vi "Reactor.vi"() -> ()   [LabVIEW 2017]
uses:
  <vilib>/Analysis/baseanly.llb/Mean (DBL).vi
  <vilib>/Utility/file.llb/Read Delimited Spreadsheet (DBL).vi
  <vilib>/Analysis/NI_AALBase.lvlib
panel:
  in  "Flow Data?":bool=TRUE
  in  "error in (no error)":errorcluster
  in  "CTAH Set Point":sgl format="%.1f"
  in  "Mode":string(combo)
  out "Server OK":bool
  out "System Time [s]":sgl
  out "Power Output":sgl(graph)
  out "Frequency [Hz]":sgl(slide) scale=0.0..60.0
  out "Frequency [Hz]":sgl(slide) scale=0.0..60.0
  out "Frequency [Hz]":sgl(knob) scale=0.0..45.0
  out "Power [W]":sgl(slide) caption="Power Output [W]" scale=0.0..10000.0
  in  "Desired Power [W]":dbl min=0.0 max=10000.0 step=1.0 format="%.1f"
  out "WT-10":sgl format="%.1f"
  out "BT-11":sgl format="%.1f"
  out "BT-12":sgl format="%.1f"
  out "WT-13":sgl format="%.1f"
  out "CX-10":dbl format="%.1f"
  out "CX-11":dbl format="%.1f"
  out "WT-20":sgl format="%.1f"
  out "BT-21":sgl format="%.1f"
  out "WT-22":sgl format="%.1f"
  out "BT-23":sgl format="%.1f"
  out "WT-24":sgl format="%.1f"
  out "BT-25":sgl format="%.1f"
  out "WT-26":sgl format="%.1f"
  out "BT-27":sgl format="%.1f"
  out "WT-28":sgl format="%.1f"
  out "BT-29":sgl format="%.1f"
  out "BT-30":sgl format="%.1f"
  out "WT-31":sgl format="%.1f"
  out "BT-32":sgl format="%.1f"
  out "WT-33":sgl format="%.1f"
  out "BT-34":sgl format="%.1f"
  out "WT-35":sgl format="%.1f"
  out "WT-40":sgl format="%.1f"
  out "BT-41":sgl format="%.1f"
  out "WT-42":sgl format="%.1f"
  out "BT-43":sgl format="%.1f"
  out "BT-60":sgl format="%.1f"
  out "WT-61":sgl format="%.1f"
  out "WT-62":sgl format="%.1f"
  out "BT-63":sgl format="%.1f"
  out "WT-64":sgl format="%.1f"
  out "BT-65":sgl format="%.1f"
  out "BT-66":sgl format="%.1f"
  out "WT-67":sgl format="%.1f"
  out "ST-10":sgl format="%.1f"
  out "ST-11":sgl format="%.1f"
  out "ST-12":sgl[](array[numeric]) format="%.1f"
  out "ST-13":sgl format="%.1f"
  out "ST-14":sgl[](array[numeric]) format="%.1f"
  out "AT-01":sgl format="%.1f"
  out "AT-02":sgl format="%.1f"
  in  "Power Output On":bool
  in  "ACTIVATE - CTAH":bool
  in  "ACTIVATE - TCHX":bool
  in  "TCHX Frequency [Hz]":sgl min=0 max=60 step=0.1 format="%.1f"
  in  "ACTIVATE - PUMP":bool
  in  "Pump Frequency [Hz]":sgl min=0 max=45 step=0.1 format="%.1f"
  out "DHX Primary Flow\n\n\nFM-20 [kg/s]":sgl format="%.3f"
  out "Bypass Flow\n\n\nFM-30 [kg/s]":sgl format="%.3f"
  out "Primary Flow\n\n\nFM-40 [kg/s]":sgl format="%.3f"
  out "DRACS Flow\n\n\nFM-60 [kg/s]":sgl format="%.3f"
  out "System Safe":bool
  in  "Exit Profile":bool
  in  "Select Operation Mode":T1(ring) caption="Select Operation Mode2"
  out "System Loop Time (ms)":u32
  in  "Load Power Profile":bool
  in  "Dyn. Power Profile File":path
  out "CTAH Temperatures":cluster{"CTAH Outlet":dbl, "CTAH Inlet":dbl}(graph)
  out "CTAH Outlet":dbl format="%0.2f"
  out "CTAH Inlet":dbl format="%0.2f"
  out "Core Temperatures":cluster{"Heater Inlet":dbl, "Heater Outlet":dbl}(graph)
  out "Heater Outlet":dbl format="%0.2f"
  out "Heater Inlet":dbl format="%0.2f"
  out "Profile Step":i32
  out "Power Input Signal [W]":dbl
  out "Output Current 2 [A]":dbl
  out "Output Voltage 2 [V]":dbl
  out "Output Current 1 [A]":dbl
  out "Output Voltage 1 [V]":dbl
  out "Loop Period [ms]":i64
  in  "Pump Operation Mode":i32(listbox)
  in  "TCHX Operation Mode":i32(listbox)
  in  "CTAH Operation Mode":i32(listbox)
  in  "Stop Reactor Interface":bool
  # "DRACS"
  # "PRIMARY"
  # "HOT DRACS"
  # "TCHX"
  # "HOT LEG"
  # "DHX TOP"
  # "N"
  # "COLD DRACS"
  # "DHX"
  # "E"
  # "S"
  # "W"
  # "BYPASS"
  # "N"
  # "CTAH"
  # "SE"
  # "SW"
  # "HEATER"
  # "DHX BOTTOM"
  # "COLD LEG"
  # "PUMP"
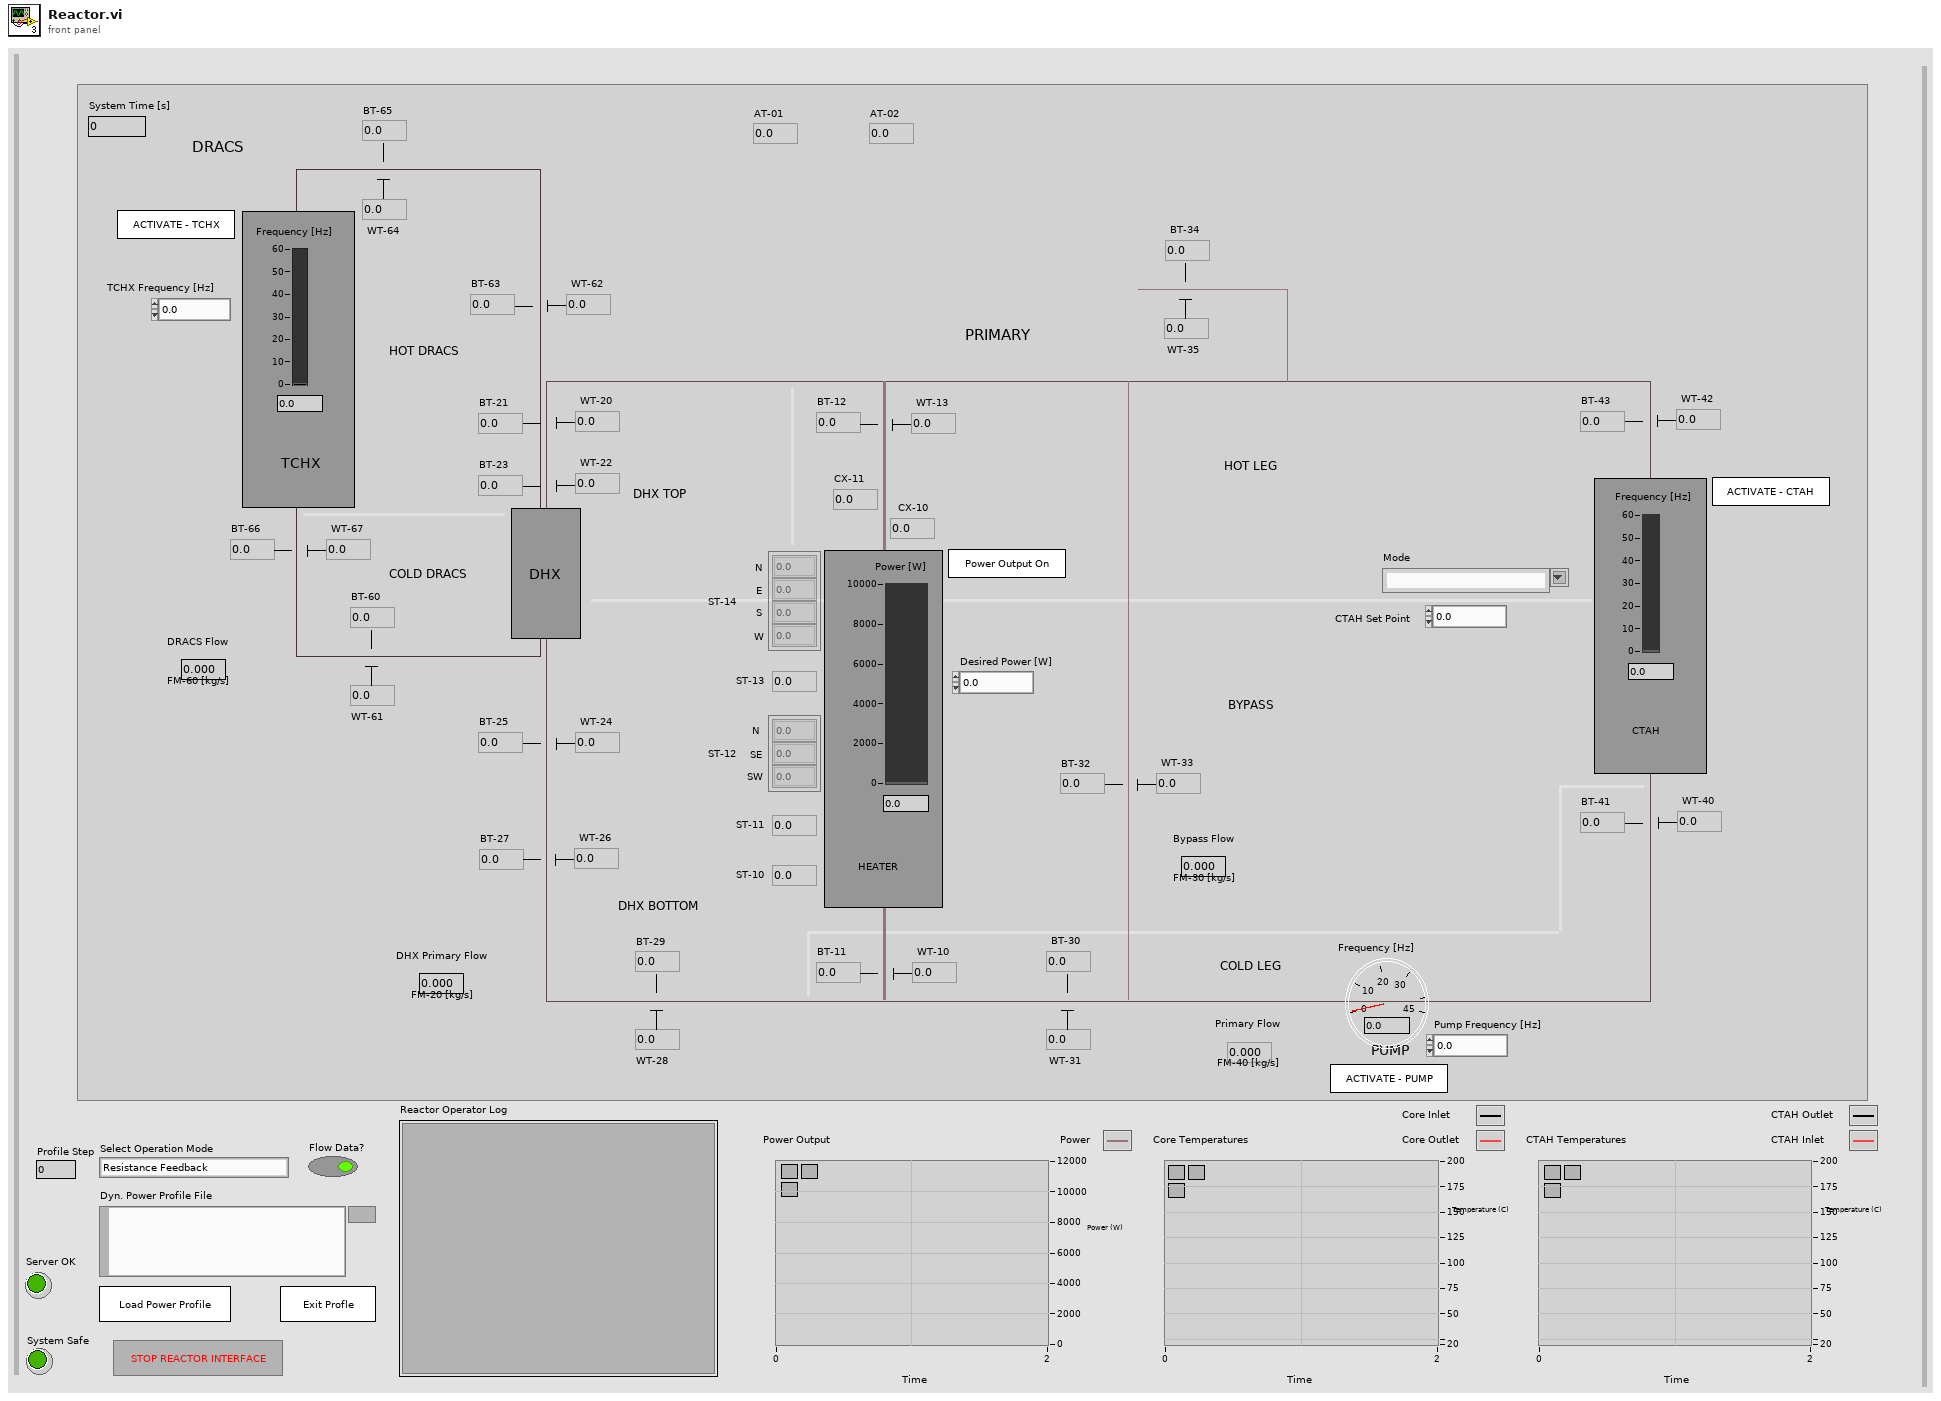
[diagram p1: front panel]
types:
  T1 = enum16{"Resistance Feedback", "Power Profile Input", "Resistance Feedback_Analog", "Power Profile Input_Analog", "Shutdown"}
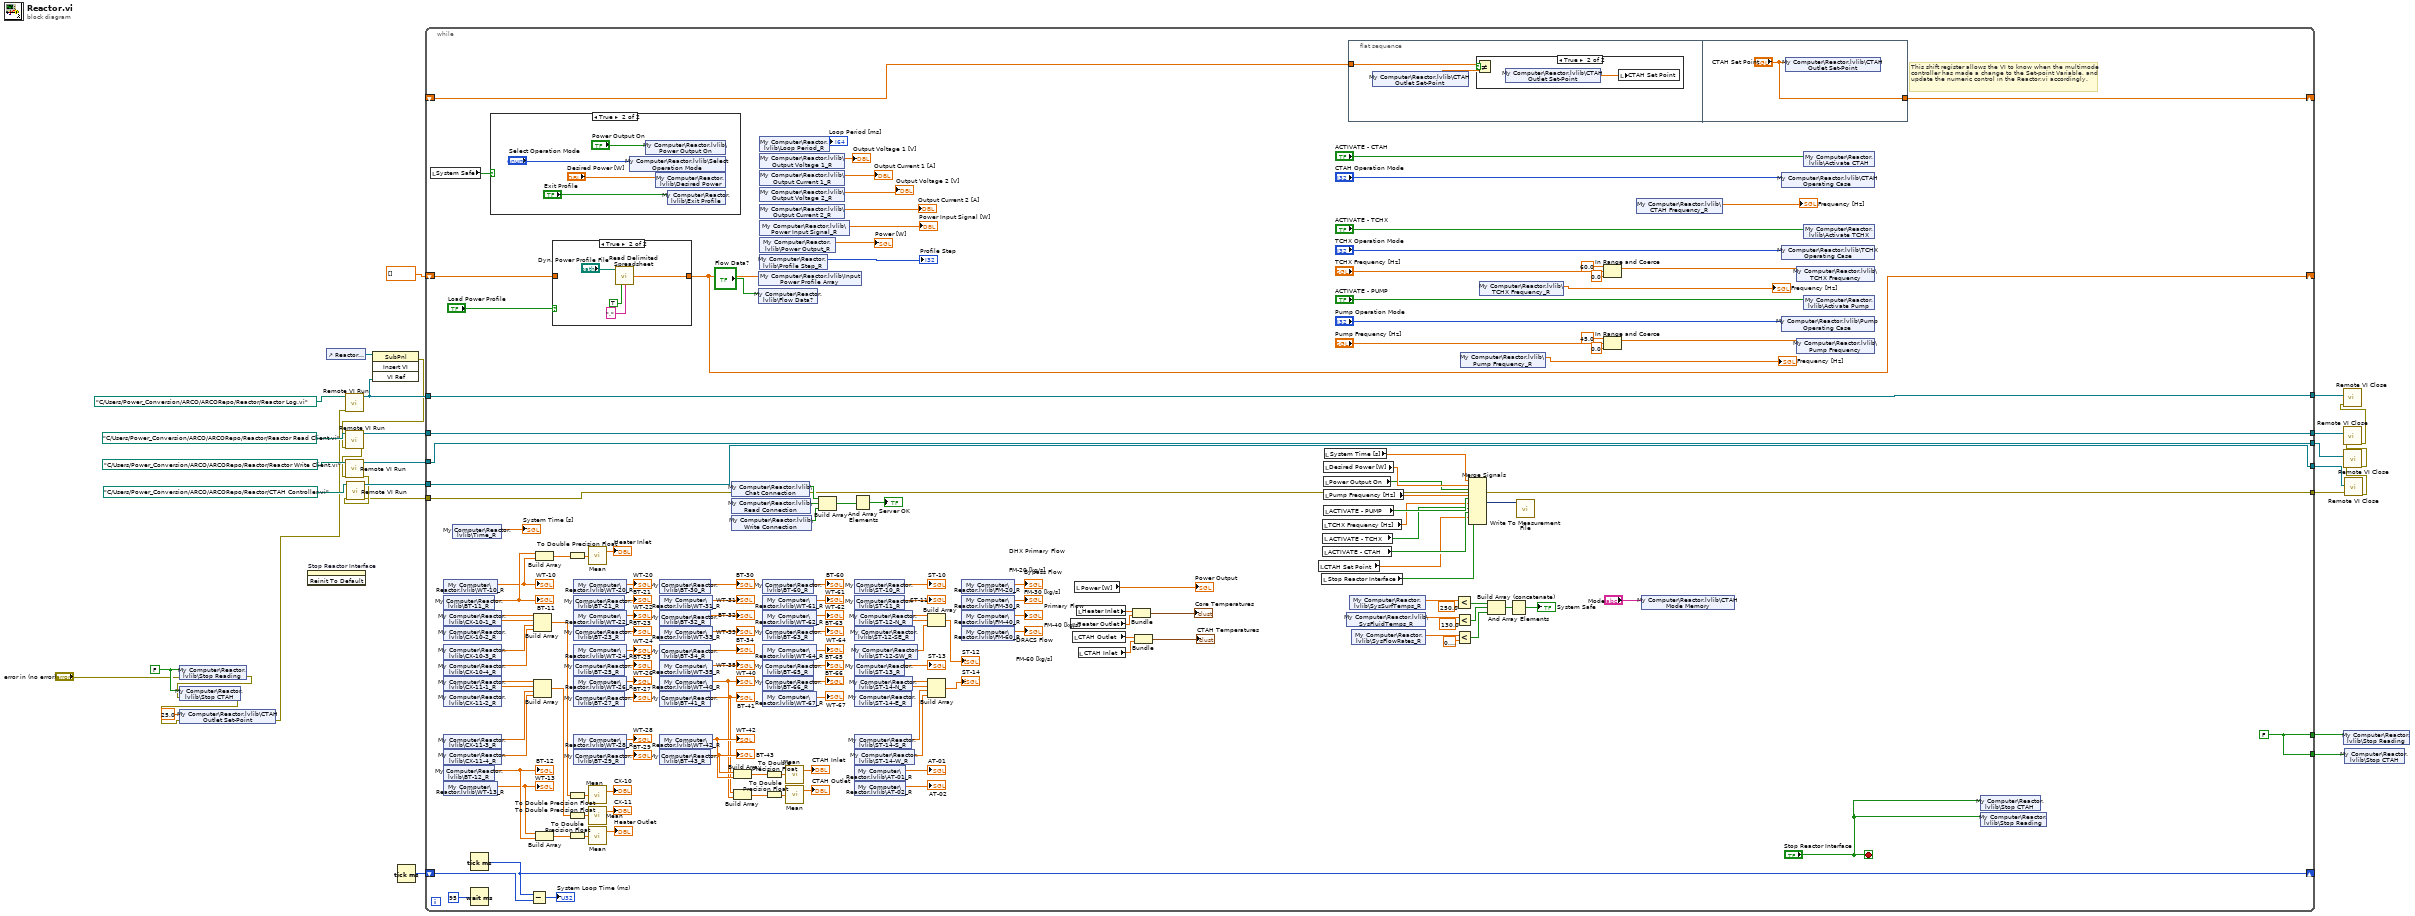
[diagram p0: block diagram]
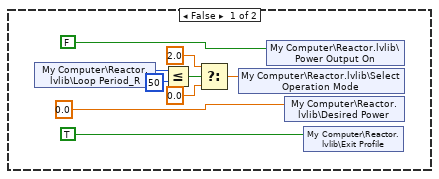
[diagram p3: hidden frame]
diagram:
  w14 = FALSE
  n1 = shared-variable "My Computer\\Reactor.lvlib\\Stop Reading"(w14, error in="error in (no error)") -> (error out=w12:errorcluster)
  n2 = shared-variable "My Computer\\Reactor.lvlib\\Stop CTAH"(w14, error in=w12) -> (error out=w11:errorcluster)
  n3 = shared-variable "My Computer\\Reactor.lvlib\\CTAH Outlet Set-Point"(25.0 ("CTAH Outlet Set-Point"), error in=w11) -> (error out=w9:errorcluster)
  n4 = invoke on="Stop Reactor Interface" class="Bool (strict)" method="Reinit To Default"() -> ()  [unwired: 3 in, 3 out]
  n5 = control-ref of="Reactor Operator Log"() -> (w25:refnum<vi>)
  n6 = call "Remote VI Run.vi"("error in (no error)"=w9, "VI Path"=path "C:/Users/Power_Conversion/ARCO/ARCORepo/Reactor/Reactor Log.vi" ("vi path")) -> ("VI Reference"=w29:refnum<vi>)  [unwired: 8 in, 1 out]
  n7 = invoke on="Invoke Node" class="SubPnl" method="Insert VI"(reference=w25, "VI Ref"=w29) -> (error out=w1:errorcluster)  [unwired: 2 in, 3 out]
  n8 = call "Remote VI Run.vi"("error in (no error)"=w1, "VI Path"=path "C:/Users/Power_Conversion/ARCO/ARCORepo/Reactor/Reactor Read Client.vi" ("vi path")) -> ("error out"=w8:errorcluster, "VI Reference"=w27:refnum<vi>)  [unwired: 8 in]
  n9 = call "Remote VI Run.vi"("error in (no error)"=w8, "VI Path"=path "C:/Users/Power_Conversion/ARCO/ARCORepo/Reactor/Reactor Write Client.vi" ("vi path")) -> ("error out"=w7:errorcluster, "VI Reference"=w20:refnum<vi>)  [unwired: 8 in]
  n10 = call "Remote VI Run.vi"("error in (no error)"=w7, "VI Path"=path "C:/Users/Power_Conversion/ARCO/ARCORepo/Reactor/CTAH Controller.vi" ("vi path")) -> ("error out"=w6:errorcluster, "VI Reference"=w17:refnum<vi>)  [unwired: 8 in]
  n11 = Tick Count (ms)() -> (millisecond timer value=w30:u32)
  n12 = while {
    shift-right: [w86] -> _
    shift-left: dbl[] [] ("Input Power Profile Array") -> [w87]
    shift-right: [w84] -> _
    shift-left: w30 -> [w85]
    tunnel: w29 -> [w66]
    tunnel: [w66] -> w28
    tunnel: w27 -> [w65]
    tunnel: [w65] -> w26
    tunnel: [w36] -> w24
    tunnel: w20 -> [w40]
    tunnel: [w40] -> w19
    tunnel: w17 -> [w37]
    tunnel: [w37] -> w16
    tunnel: [w36] -> w15
    shift-right: [w35] -> _
    shift-left: _ -> [w34]
    tunnel: w6 -> [w32]
    tunnel: [w32] -> w5
    stop <- "Stop Reactor Interface" stop-if-true
    w36 = FALSE
    # "This shift register allows the VI to know when the multimode controller has made a change to the Set-point Variable, and update the numeric control in the Reactor.vi accordingly."
    n13 = local read "System Safe"() -> (w70:bool)
    n14 = shared-variable "My Computer\\Reactor.lvlib\\WT-10_R"() -> (w107:sgl)  [unwired: 1 in, 1 out]
    "WT-10" <- w107
    n15 = shared-variable "My Computer\\Reactor.lvlib\\BT-11_R"() -> (w108:sgl)  [unwired: 1 in, 1 out]
    "BT-11" <- w108
    n16 = shared-variable "My Computer\\Reactor.lvlib\\CX-10-1_R"() -> (w170:sgl)  [unwired: 1 in, 1 out]
    n17 = shared-variable "My Computer\\Reactor.lvlib\\CX-10-2_R"() -> (w169:sgl)  [unwired: 1 in, 1 out]
    n18 = shared-variable "My Computer\\Reactor.lvlib\\CX-10-3_R"() -> (w168:sgl)  [unwired: 1 in, 1 out]
    n19 = shared-variable "My Computer\\Reactor.lvlib\\CX-10-4_R"() -> (w167:sgl)  [unwired: 1 in, 1 out]
    n20 = shared-variable "My Computer\\Reactor.lvlib\\CX-11-1_R"() -> (w163:sgl)  [unwired: 1 in, 1 out]
    n21 = shared-variable "My Computer\\Reactor.lvlib\\CX-11-2_R"() -> (w162:sgl)  [unwired: 1 in, 1 out]
    n22 = shared-variable "My Computer\\Reactor.lvlib\\CX-11-3_R"() -> (w161:sgl)  [unwired: 1 in, 1 out]
    n23 = shared-variable "My Computer\\Reactor.lvlib\\CX-11-4_R"() -> (w160:sgl)  [unwired: 1 in, 1 out]
    n24 = shared-variable "My Computer\\Reactor.lvlib\\BT-12_R"() -> (w112:sgl)  [unwired: 1 in, 1 out]
    "BT-12" <- w112
    n25 = shared-variable "My Computer\\Reactor.lvlib\\WT-13_R"() -> (w111:sgl)  [unwired: 1 in, 1 out]
    "WT-13" <- w111
    n26 = shared-variable "My Computer\\Reactor.lvlib\\Time_R"() -> (→"System Time [s]":sgl)  [unwired: 1 in, 1 out]
    n27 = Tick Count (ms)() -> (millisecond timer value=w84:u32)
    n28 = Wait (ms)(milliseconds to wait=u32 95) -> ()  [unwired: 1 out]
    n29 = case shown="True" w70 {
      frame False {
        n30 = shared-variable "My Computer\\Reactor.lvlib\\Loop Period_R"() -> (w196:i64)  [unwired: 1 in, 1 out]
        n31 = Less Or Equal?(x=w196, y=i64 50) -> (x <= y?=w197:bool)
        n32 = Select(t=2.0, s=w197, f=0.0) -> (s? t:f=w192:dbl)
        n33 = shared-variable "My Computer\\Reactor.lvlib\\Select Operation Mode"(w192) -> ()  [unwired: 1 in, 1 out]
        n34 = shared-variable "My Computer\\Reactor.lvlib\\Power Output On"(FALSE ("Power Output On")) -> ()  [unwired: 1 in, 1 out]
        n35 = shared-variable "My Computer\\Reactor.lvlib\\Desired Power"(0.0 ("Desired Power")) -> ()  [unwired: 1 in, 1 out]
        n36 = shared-variable "My Computer\\Reactor.lvlib\\Exit Profile"(TRUE ("Exit Profile")) -> ()  [unwired: 1 in, 1 out]
      }
      frame True {
        n37 = shared-variable "My Computer\\Reactor.lvlib\\Select Operation Mode"("Select Operation Mode") -> ()  [unwired: 1 in, 1 out]
        n38 = shared-variable "My Computer\\Reactor.lvlib\\Power Output On"("Power Output On") -> ()  [unwired: 1 in, 1 out]
        n39 = shared-variable "My Computer\\Reactor.lvlib\\Desired Power"("Desired Power [W]") -> ()  [unwired: 1 in, 1 out]
        n40 = shared-variable "My Computer\\Reactor.lvlib\\Exit Profile"("Exit Profile") -> ()  [unwired: 1 in, 1 out]
      }
    }
    n41 = Subtract(x=w84, y=w85) -> (x-y=→"System Loop Time (ms)":u32)
    n42 = Build Array(w170, w169, w168, w167) -> (w166:sgl[])
    n43 = Build Array(w163, w162, w161, w160) -> (w159:sgl[])
    n44 = Build Array(w108, w107) -> (w109:sgl[])
    n45 = Build Array(w111, w112) -> (w113:sgl[])
    n46 = case shown="True" "Load Power Profile" {
      tunnel: [w205 w206] -> w86
      tunnel: w87 -> [w205 _]
      frame False {
      }
      frame True {
        n47 = call-poly <vilib>:"Read Delimited Spreadsheet.vi"("file path (dialog if empty)"="Dyn. Power Profile File", "transpose? (F)"=TRUE, "delimiter (\\t)"="," ("delimiter (\\t)")) -> ("first row"=w206:dbl[])  [unwired: 7 in, 5 out]
      }
    }
    n48 = To Double Precision Float(number=w109) -> (double precision float=w110:dbl[])
    n49 = To Double Precision Float(number=w166) -> (double precision float=w165:dbl[])
    n50 = To Double Precision Float(number=w159) -> (double precision float=w164:dbl[])
    n51 = To Double Precision Float(number=w113) -> (double precision float=w114:dbl[])
    n52 = shared-variable "My Computer\\Reactor.lvlib\\WT-20_R"() -> (→"WT-20":sgl)  [unwired: 1 in, 1 out]
    n53 = shared-variable "My Computer\\Reactor.lvlib\\BT-21_R"() -> (→"BT-21":sgl)  [unwired: 1 in, 1 out]
    n54 = shared-variable "My Computer\\Reactor.lvlib\\WT-22_R"() -> (→"WT-22":sgl)  [unwired: 1 in, 1 out]
    n55 = shared-variable "My Computer\\Reactor.lvlib\\BT-23_R"() -> (→"BT-23":sgl)  [unwired: 1 in, 1 out]
    n56 = shared-variable "My Computer\\Reactor.lvlib\\WT-24_R"() -> (→"WT-24":sgl)  [unwired: 1 in, 1 out]
    n57 = shared-variable "My Computer\\Reactor.lvlib\\BT-25_R"() -> (→"BT-25":sgl)  [unwired: 1 in, 1 out]
    n58 = shared-variable "My Computer\\Reactor.lvlib\\WT-26_R"() -> (→"WT-26":sgl)  [unwired: 1 in, 1 out]
    n59 = shared-variable "My Computer\\Reactor.lvlib\\BT-27_R"() -> (→"BT-27":sgl)  [unwired: 1 in, 1 out]
    n60 = shared-variable "My Computer\\Reactor.lvlib\\WT-28_R"() -> (→"WT-28":sgl)  [unwired: 1 in, 1 out]
    n61 = shared-variable "My Computer\\Reactor.lvlib\\BT-29_R"() -> (→"BT-29":sgl)  [unwired: 1 in, 1 out]
    n62 = call-poly <vilib>:"Mean.vi"("X"=w110) -> ("mean"=→"Heater Inlet":dbl)  [unwired: 1 out]
    n63 = call-poly <vilib>:"Mean.vi"("X"=w165) -> ("mean"=→"CX-10":dbl)  [unwired: 1 out]
    n64 = call-poly <vilib>:"Mean.vi"("X"=w164) -> ("mean"=→"CX-11":dbl)  [unwired: 1 out]
    n65 = call-poly <vilib>:"Mean.vi"("X"=w114) -> ("mean"=→"Heater Outlet":dbl)  [unwired: 1 out]
    n66 = shared-variable "My Computer\\Reactor.lvlib\\BT-30_R"() -> (→"BT-30":sgl)  [unwired: 1 in, 1 out]
    n67 = shared-variable "My Computer\\Reactor.lvlib\\WT-31_R"() -> (→"WT-31":sgl)  [unwired: 1 in, 1 out]
    n68 = shared-variable "My Computer\\Reactor.lvlib\\BT-32_R"() -> (→"BT-32":sgl)  [unwired: 1 in, 1 out]
    n69 = shared-variable "My Computer\\Reactor.lvlib\\WT-33_R"() -> (→"WT-33":sgl)  [unwired: 1 in, 1 out]
    n70 = shared-variable "My Computer\\Reactor.lvlib\\BT-34_R"() -> (→"BT-34":sgl)  [unwired: 1 in, 1 out]
    n71 = shared-variable "My Computer\\Reactor.lvlib\\WT-35_R"() -> (→"WT-35":sgl)  [unwired: 1 in, 1 out]
    n72 = shared-variable "My Computer\\Reactor.lvlib\\WT-40_R"() -> (w93:sgl)  [unwired: 1 in, 1 out]
    "WT-40" <- w93
    n73 = shared-variable "My Computer\\Reactor.lvlib\\BT-41_R"() -> (w92:sgl)  [unwired: 1 in, 1 out]
    "BT-41" <- w92
    n74 = shared-variable "My Computer\\Reactor.lvlib\\WT-42_R"() -> (w95:sgl)  [unwired: 1 in, 1 out]
    "WT-42" <- w95
    n75 = shared-variable "My Computer\\Reactor.lvlib\\BT-43_R"() -> (w94:sgl)  [unwired: 1 in, 1 out]
    "BT-43" <- w94
    n76 = shared-variable "My Computer\\Reactor.lvlib\\Chat Connection"() -> (w64:bool)  [unwired: 1 in, 1 out]
    n77 = shared-variable "My Computer\\Reactor.lvlib\\Read Connection"() -> (w63:bool)  [unwired: 1 in, 1 out]
    n78 = shared-variable "My Computer\\Reactor.lvlib\\Write Connection"() -> (w39:bool)  [unwired: 1 in, 1 out]
    n79 = Build Array(w94, w95) -> (w100:sgl[])
    n80 = Build Array(w92, w93) -> (w97:sgl[])
    n81 = shared-variable "My Computer\\Reactor.lvlib\\Input Power Profile Array"(w86) -> ()  [unwired: 1 in, 1 out]
    n82 = shared-variable "My Computer\\Reactor.lvlib\\Flow Data?"("Flow Data?") -> ()  [unwired: 1 in, 1 out]
    n83 = shared-variable "My Computer\\Reactor.lvlib\\Loop Period_R"() -> (→"Loop Period [ms]":i64)  [unwired: 1 in, 1 out]
    n84 = shared-variable "My Computer\\Reactor.lvlib\\Output Voltage 1_R"() -> (→"Output Voltage 1 [V]":dbl)  [unwired: 1 in, 1 out]
    n85 = shared-variable "My Computer\\Reactor.lvlib\\Output Current 1_R"() -> (→"Output Current 1 [A]":dbl)  [unwired: 1 in, 1 out]
    n86 = shared-variable "My Computer\\Reactor.lvlib\\Output Voltage 2_R"() -> (→"Output Voltage 2 [V]":dbl)  [unwired: 1 in, 1 out]
    n87 = shared-variable "My Computer\\Reactor.lvlib\\Output Current 2_R"() -> (→"Output Current 2 [A]":dbl)  [unwired: 1 in, 1 out]
    n88 = shared-variable "My Computer\\Reactor.lvlib\\Power Input Signal_R"() -> (→"Power Input Signal [W]":sgl)  [unwired: 1 in, 1 out]
    n89 = shared-variable "My Computer\\Reactor.lvlib\\Power Output_R"() -> (→"Power [W]":sgl)  [unwired: 1 in, 1 out]
    n90 = shared-variable "My Computer\\Reactor.lvlib\\Profile Step_R"() -> (→"Profile Step":i32)  [unwired: 1 in, 1 out]
    n91 = shared-variable "My Computer\\Reactor.lvlib\\BT-60_R"() -> (→"BT-60":sgl)  [unwired: 1 in, 1 out]
    n92 = shared-variable "My Computer\\Reactor.lvlib\\WT-61_R"() -> (→"WT-61":sgl)  [unwired: 1 in, 1 out]
    n93 = shared-variable "My Computer\\Reactor.lvlib\\WT-62_R"() -> (→"WT-62":sgl)  [unwired: 1 in, 1 out]
    n94 = shared-variable "My Computer\\Reactor.lvlib\\BT-63_R"() -> (→"BT-63":sgl)  [unwired: 1 in, 1 out]
    n95 = shared-variable "My Computer\\Reactor.lvlib\\WT-64_R"() -> (→"WT-64":sgl)  [unwired: 1 in, 1 out]
    n96 = shared-variable "My Computer\\Reactor.lvlib\\BT-65_R"() -> (→"BT-65":sgl)  [unwired: 1 in, 1 out]
    n97 = shared-variable "My Computer\\Reactor.lvlib\\BT-66_R"() -> (→"BT-66":sgl)  [unwired: 1 in, 1 out]
    n98 = shared-variable "My Computer\\Reactor.lvlib\\WT-67_R"() -> (→"WT-67":sgl)  [unwired: 1 in, 1 out]
    n99 = To Double Precision Float(number=w100) -> (double precision float=w101:dbl[])
    n100 = To Double Precision Float(number=w97) -> (double precision float=w98:dbl[])
    n101 = call-poly <vilib>:"Mean.vi"("X"=w101) -> ("mean"=→"CTAH Inlet":dbl)  [unwired: 1 out]
    n102 = call-poly <vilib>:"Mean.vi"("X"=w98) -> ("mean"=→"CTAH Outlet":dbl)  [unwired: 1 out]
    n103 = Build Array(w64, w63, w39) -> (w62:bool[])
    n104 = And Array Elements(Boolean array=w62) -> (logical AND=→"Server OK":bool)
    n105 = shared-variable "My Computer\\Reactor.lvlib\\ST-10_R"() -> (→"ST-10":sgl)  [unwired: 1 in, 1 out]
    n106 = shared-variable "My Computer\\Reactor.lvlib\\ST-11_R"() -> (→"ST-11":sgl)  [unwired: 1 in, 1 out]
    n107 = shared-variable "My Computer\\Reactor.lvlib\\ST-12-N_R"() -> (w130:sgl)  [unwired: 1 in, 1 out]
    n108 = shared-variable "My Computer\\Reactor.lvlib\\ST-12-SE_R"() -> (w129:sgl)  [unwired: 1 in, 1 out]
    n109 = shared-variable "My Computer\\Reactor.lvlib\\ST-12-SW_R"() -> (w128:sgl)  [unwired: 1 in, 1 out]
    n110 = shared-variable "My Computer\\Reactor.lvlib\\ST-13_R"() -> (→"ST-13":sgl)  [unwired: 1 in, 1 out]
    n111 = shared-variable "My Computer\\Reactor.lvlib\\ST-14-N_R"() -> (w125:sgl)  [unwired: 1 in, 1 out]
    n112 = shared-variable "My Computer\\Reactor.lvlib\\ST-14-E_R"() -> (w124:sgl)  [unwired: 1 in, 1 out]
    n113 = shared-variable "My Computer\\Reactor.lvlib\\ST-14-S_R"() -> (w123:sgl)  [unwired: 1 in, 1 out]
    n114 = shared-variable "My Computer\\Reactor.lvlib\\ST-14-W_R"() -> (w122:sgl)  [unwired: 1 in, 1 out]
    n115 = shared-variable "My Computer\\Reactor.lvlib\\AT-01_R"() -> (→"AT-01":sgl)  [unwired: 1 in, 1 out]
    n116 = shared-variable "My Computer\\Reactor.lvlib\\AT-02_R"() -> (→"AT-02":sgl)  [unwired: 1 in, 1 out]
    n117 = Build Array(w130, w129, w128) -> (→"ST-12":sgl[])
    n118 = Build Array(w125, w124, w123, w122) -> (→"ST-14":sgl[])
    n119 = shared-variable "My Computer\\Reactor.lvlib\\FM-20_R"() -> (→"DHX Primary Flow\n\n\nFM-20 [kg/s]":sgl)  [unwired: 1 in, 1 out]
    n120 = shared-variable "My Computer\\Reactor.lvlib\\FM-30_R"() -> (→"Bypass Flow\n\n\nFM-30 [kg/s]":sgl)  [unwired: 1 in, 1 out]
    n121 = shared-variable "My Computer\\Reactor.lvlib\\FM-40_R"() -> (→"Primary Flow\n\n\nFM-40 [kg/s]":sgl)  [unwired: 1 in, 1 out]
    n122 = shared-variable "My Computer\\Reactor.lvlib\\FM-60_R"() -> (→"DRACS Flow\n\n\nFM-60 [kg/s]":sgl)  [unwired: 1 in, 1 out]
    n123 = local read "Heater Outlet"() -> (w102:dbl)
    n124 = local read "CTAH Outlet"() -> (w90:dbl)
    n125 = local read "Power [W]"() -> (→"Power Output":sgl)
    n126 = local read "Heater Inlet"() -> (w103:dbl)
    n127 = local read "CTAH Inlet"() -> (w89:dbl)
    n128 = Bundle("Heater Inlet"=w103, "Heater Outlet"=w102) -> (→"Core Temperatures":cluster{"Heater Inlet":dbl, "Heater Outlet":dbl})  [unwired: 1 in]
    n129 = Bundle("CTAH Outlet"=w90, "CTAH Inlet"=w89) -> (→"CTAH Temperatures":cluster{"CTAH Outlet":dbl, "CTAH Inlet":dbl})  [unwired: 1 in]
    n130 = local read "CTAH Set Point"() -> (w43:sgl)
    n131 = local read "Stop Reactor Interface"() -> (w42:bool)
    n132 = local read "TCHX Frequency [Hz]"() -> (w46:sgl)
    n133 = local read "ACTIVATE - CTAH"() -> (w44:bool)
    n134 = local read "ACTIVATE - TCHX"() -> (w45:bool)
    n135 = local read "Desired Power [W]"() -> (w50:dbl)
    n136 = local read "Power Output On"() -> (w49:bool)
    n137 = local read "Pump Frequency [Hz]"() -> (w48:sgl)
    n138 = local read "ACTIVATE - PUMP"() -> (w47:bool)
    n139 = local read "System Time [s]"() -> (w51:sgl)
    n140 = shared-variable "My Computer\\Reactor.lvlib\\SysFluidTemps_R"() -> (w76:sgl[])  [unwired: 1 in, 1 out]
    n141 = flat-sequence {
      tunnel: w34 -> [w187]
      tunnel: ["CTAH Set Point"] -> w35
      frame #0 {
        n142 = shared-variable "My Computer\\Reactor.lvlib\\CTAH Outlet Set-Point"() -> (w188:dbl)  [unwired: 1 in, 1 out]
        n143 = Not Equal?(x=w187, y=w188) -> (x != y?=w189:bool)
        n144 = case shown="True" w189 {
          frame False {
          }
          frame True {
            n145 = shared-variable "My Computer\\Reactor.lvlib\\CTAH Outlet Set-Point"() -> (w190:dbl)  [unwired: 1 in, 1 out]
            n146 = local write "CTAH Set Point"(w190) -> ()
          }
        }
      }
      frame #1 {
        n147 = shared-variable "My Computer\\Reactor.lvlib\\CTAH Outlet Set-Point"("CTAH Set Point") -> ()  [unwired: 1 in, 1 out]
      }
    }
    n148 = shared-variable "My Computer\\Reactor.lvlib\\SysSurfTemps_R"() -> (w78:sgl[])  [unwired: 1 in, 1 out]
    n149 = shared-variable "My Computer\\Reactor.lvlib\\SysFlowRates_R"() -> (w74:sgl[])  [unwired: 1 in, 1 out]
    n150 = Less?(x=w78, y=sgl 250.0) -> (x < y?=w80:bool[])
    n151 = Less?(x=w76, y=sgl 130.0) -> (x < y?=w73:bool[])
    n152 = Less?(x=w74, y=sgl 0.2) -> (x < y?=w72:bool[])
    n153 = shared-variable "My Computer\\Reactor.lvlib\\Pump Frequency_R"() -> (→"Frequency [Hz]":sgl)  [unwired: 1 in, 1 out]
    n154 = Merge Signals(w51, w50, w49, w48, w47, w46, w45, w44, w43, w42) -> (w52:dynamicdata)
    n155 = shared-variable "My Computer\\Reactor.lvlib\\TCHX Frequency_R"() -> (→"Frequency [Hz]":sgl)  [unwired: 1 in, 1 out]
    n156 = Build Array (concatenate)(w80, w73, w72) -> (w81:bool[])
    n157 = And Array Elements(Boolean array=w81) -> (logical AND=→"System Safe":bool)
    n158 = call "Write To Measurement File"("Signals"=w52) -> ()  [unwired: 16 in, 3 out]
    n159 = In Range and Coerce(upper limit=sgl 60.0, x="TCHX Frequency [Hz]", lower limit=sgl 0.0) -> (coerced(x)=w56:sgl)  [unwired: 1 out]
    n160 = In Range and Coerce(upper limit=sgl 45.0, x="Pump Frequency [Hz]", lower limit=sgl 0.0) -> (coerced(x)=w55:sgl)  [unwired: 1 out]
    n161 = shared-variable "My Computer\\Reactor.lvlib\\CTAH Frequency_R"() -> (→"Frequency [Hz]":sgl)  [unwired: 1 in, 1 out]
    n162 = shared-variable "My Computer\\Reactor.lvlib\\CTAH Mode Memory"("Mode") -> ()  [unwired: 1 in, 1 out]
    n163 = shared-variable "My Computer\\Reactor.lvlib\\CTAH Operating Case"("CTAH Operation Mode") -> ()  [unwired: 1 in, 1 out]
    n164 = shared-variable "My Computer\\Reactor.lvlib\\Pump Operating Case"("Pump Operation Mode") -> ()  [unwired: 1 in, 1 out]
    n165 = shared-variable "My Computer\\Reactor.lvlib\\TCHX Operating Case"("TCHX Operation Mode") -> ()  [unwired: 1 in, 1 out]
    n166 = shared-variable "My Computer\\Reactor.lvlib\\Pump Frequency"(w55) -> ()  [unwired: 1 in, 1 out]
    n167 = shared-variable "My Computer\\Reactor.lvlib\\TCHX Frequency"(w56) -> ()  [unwired: 1 in, 1 out]
    n168 = shared-variable "My Computer\\Reactor.lvlib\\Activate CTAH"("ACTIVATE - CTAH") -> ()  [unwired: 1 in, 1 out]
    n169 = shared-variable "My Computer\\Reactor.lvlib\\Activate Pump"("ACTIVATE - PUMP") -> ()  [unwired: 1 in, 1 out]
    n170 = shared-variable "My Computer\\Reactor.lvlib\\Activate TCHX"("ACTIVATE - TCHX") -> ()  [unwired: 1 in, 1 out]
    n171 = shared-variable "My Computer\\Reactor.lvlib\\Stop CTAH"("Stop Reactor Interface") -> ()  [unwired: 1 in, 1 out]
    n172 = shared-variable "My Computer\\Reactor.lvlib\\Stop Reading"("Stop Reactor Interface") -> ()  [unwired: 1 in, 1 out]
  }
  n173 = shared-variable "My Computer\\Reactor.lvlib\\Stop Reading"(w24) -> ()  [unwired: 1 in, 1 out]
  n174 = call "Remote VI Close.vi"("error in (no error)"=w5, "reference"=w16) -> ("error out"=w4:errorcluster)  [unwired: 8 in, 1 out]
  n175 = call "Remote VI Close.vi"("error in (no error)"=w4, "reference"=w19) -> ("error out"=w3:errorcluster)  [unwired: 8 in, 1 out]
  n176 = call "Remote VI Close.vi"("error in (no error)"=w3, "reference"=w26) -> ("error out"=w2:errorcluster)  [unwired: 8 in, 1 out]
  n177 = call "Remote VI Close.vi"("error in (no error)"=w2, "reference"=w28) -> ()  [unwired: 8 in, 2 out]
  n178 = shared-variable "My Computer\\Reactor.lvlib\\Stop CTAH"(w15) -> ()  [unwired: 1 in, 1 out]
